vi "Act.vi"(8 "error in (no error)":errorcluster, 9 "VI Refnum in":refnum<vi>, 10 "Flex Msg type":refnum<class "Flex Msg.lvclass">, 11 "Manual Edit in":refnum<class "Manual Edit.lvclass">) -> (0 "error out":errorcluster, 1 "Await user action?":bool, 3 "Manual Edit out":refnum<class "Manual Edit.lvclass">)   [LabVIEW 2020, in "Msg.lvlib" / "Manual Edit.lvclass"]
doc: "This implementation inserts the VI in a subpanel and then waits for user action."
uses:
  Manual Edit.lvclass
  Flex Msg.lvclass
  Manual Edit.lvclass/Manual Edit.ctl
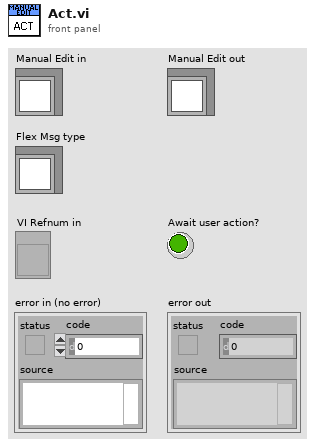
[diagram p1: front panel]
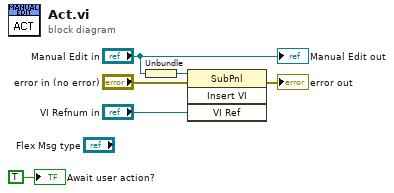
[diagram p0: block diagram]
diagram:
  n1 = Unbundle("Manual Edit in") -> (w4:refnum<vi>)
  n2 = invoke class="SubPnl" method="Insert VI"(reference=w4, error in="error in (no error)", "VI Ref"="VI Refnum in") -> (error out=→"error out":errorcluster)  [unwired: 1 in, 3 out]
  "Manual Edit out" <- "Manual Edit in"
  "Await user action?" <- TRUE ("Await user action?")
